vi "escape characters for javascript.vi"(5 "String (\"\")":string) -> (2 "escaped String":string)   [LabVIEW 2011]
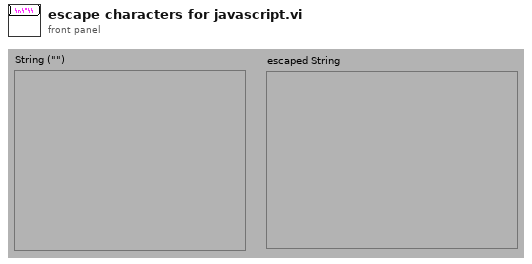
[diagram p1: front panel]
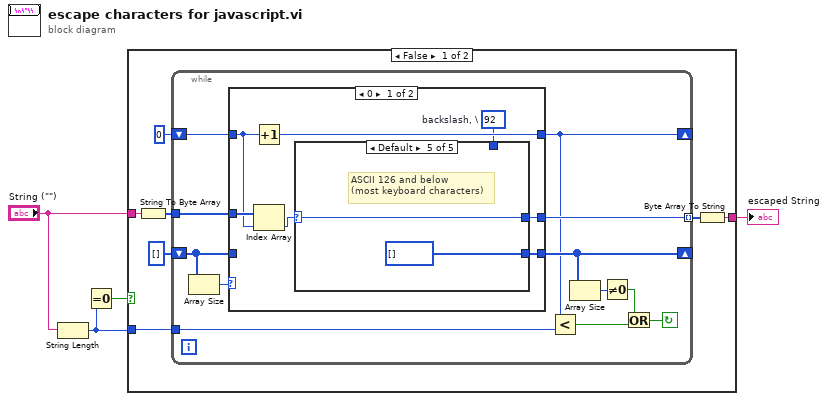
[diagram p0: block diagram]
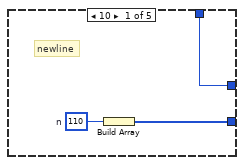
[diagram p2: hidden frame]
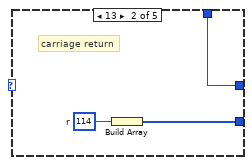
[diagram p3: hidden frame]
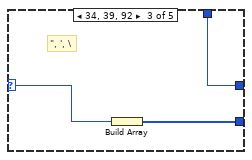
[diagram p4: hidden frame]
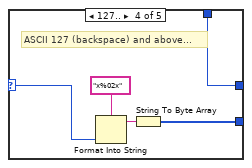
[diagram p5: hidden frame]
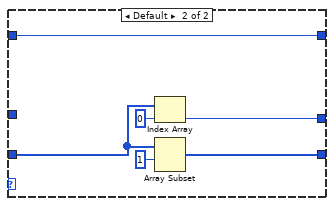
[diagram p6: hidden frame]
diagram:
  n1 = String Length(string="String (\"\")") -> (length=w2:i32)
  n2 = Equal To 0?(x=w2) -> (x = 0?=w1:bool)
  n3 = case shown="False" w1 {
    tunnel: [w7 w53] -> w4
    tunnel: "String (\"\")" -> [w6 w53]
    tunnel: w2 -> [w5 _]
    frame False {
      n4 = String To Byte Array(string=w6) -> (unsigned byte array=w9:u8[])
      n5 = while {
        tunnel: w5 -> [w19]
        shift-left: 0 ("offset past match") -> [w13]
        shift-right: [w12] -> _
        tunnel: [w21] -> w8 mode=indexing
        tunnel: w9 -> [w20]
        shift-left: u8[] [] ("Array Constant") -> [w22]
        shift-right: [w15] -> _
        stop <- w14 continue-if-true
        n6 = Array Size(array=w22) -> (size(s)=w23:i32)
        n7 = case shown="0" w23 {
          tunnel: w22 -> [_ w52]
          tunnel: [w26 w47] -> w15
          tunnel: [w28 w49] -> w21
          tunnel: w20 -> [w30 _]
          tunnel: w13 -> [w25 w48]
          tunnel: [w27 w48] -> w12
          frame 0 {
            w24 = u8 92  # backslash, \
            n8 = Increment(x=w25) -> (x+1=w27:i32)
            n9 = Index Array(array=w30, index=w25) -> (element=w29:u8)
            n10 = case shown="Default" w29 {
              selector: w29 -> [_ _ w39 w43 w46]
              tunnel: [w32 w35 w37 w40 w46] -> w28
              tunnel: [w33 w36 w38 w42 u8[] [] ("Array Constant")] -> w26
              tunnel: w24 -> [w32 w35 w37 w40 _]
              frame 10 {
                w31 = u8 110  # n
                # "newline"
                n11 = Build Array(w31) -> (w33:u8[])
              }
              frame 13 {
                w34 = u8 114  # r
                # "carriage return"
                n12 = Build Array(w34) -> (w36:u8[])
              }
              frame 34, 39, 92 {
                # "\", ', \\"
                n13 = Build Array(w39) -> (w38:u8[])
              }
              frame 127.. {
                # "ASCII 127 (backspace) and above..."
                n14 = Format Into String(format string="x%02x", w43) -> (resulting string=w41:string)  [unwired: 2 in, 1 out]
                n15 = String To Byte Array(string=w41) -> (unsigned byte array=w42:u8[])
              }
              frame Default {
                # "ASCII 126 and below\n(most keyboard characters)"
              }
            }
          }
          frame Default {
            n16 = Index Array(array=w52, index=0 ("Index")) -> (element=w49:u8)
            n17 = Array Subset(array=w52, index=1 ("Array Index")) -> (w47:u8[])  [unwired: 1 in]
          }
        }
        n18 = Less?(x=w12, y=w19) -> (x < y?=w16:bool)
        n19 = Array Size(array=w15) -> (size(s)=w17:i32)
        n20 = Not Equal To 0?(x=w17) -> (x != 0?=w18:bool)
        n21 = Or(x=w18, y=w16) -> (x .or. y?=w14:bool)
      }
      n22 = Byte Array To String(unsigned byte array=w8) -> (string=w7:string)
    }
    frame True {
    }
  }
  "escaped String" <- w4
